vi "Create DataBase.vi"(8 "error in (no error)":errorcluster, 11 "数据库名称":string) -> (0 "error out":errorcluster, 3 "connection reference":T1)   [LabVIEW 2014]
uses:
  <vilib>/addons/database/NI_Database_API.lvlib
  <vilib>/addons/database/Connection.llb/DB Tools Open Connec (String).vi
  <vilib>/addons/database/Connection.llb/Conn ObjectReference.ctl
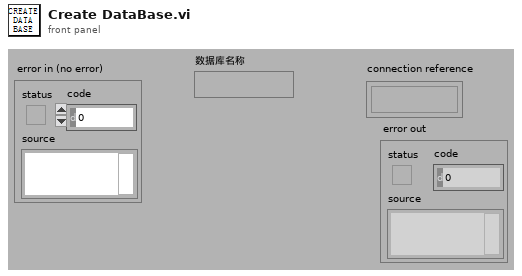
[diagram p1: front panel]
types:
  T1 = typedef "NI_Database_API.lvlib/Conn ObjectReference.ctl" = refnum<k1>
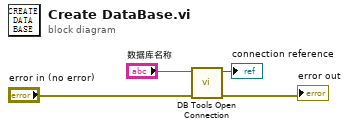
[diagram p0: block diagram]
diagram:
  n1 = call-poly <vilib>:"DB Tools Open Connection.vi"("error in (no error)"="error in (no error)", "connection information"="数据库名称") -> ("error out"=→"error out":errorcluster, "connection reference"=→"connection reference":T1)  [unwired: 6 in]
